vi "Two Color Cal Wait New Frame.vi"(0 "Notifier Name":string, 11 "Error In":errorcluster, 13 "Frames to Wait":u32) -> (15 "Error Out":errorcluster)   [LabVIEW 2016]
uses:
  Device Library/Cameras/Camera Controls/Generic Camera Actions.ctl
  Device Library/Cameras/Camera Controls/Camera IMAQ Key Info.ctl
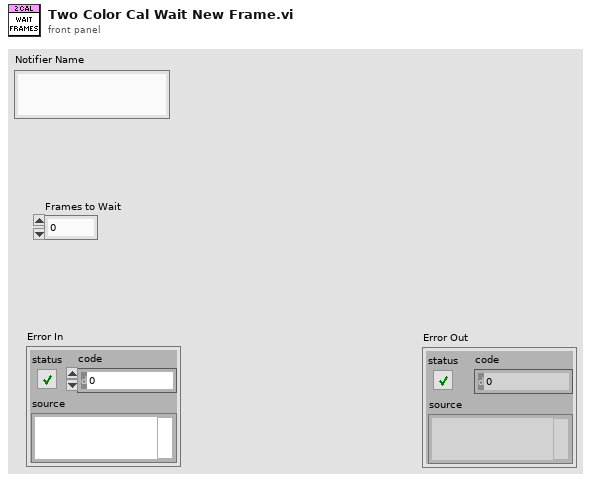
[diagram p1: front panel]
types:
  T1 = typedef "Generic Camera Actions.ctl" = enum16{"Status", "Live Preview", "Capture", "Abort", "Set Exposure Time (s)", "Get Exposure Time (s)", "Record Settings", "Set ROI", "Get ROI", "Defect Correction On/Off", "Cooler On/Off", "Fan On/Off", "Quti"}
  T2 = typedef "IMAQ Image.ctl" = refnum<image>
  T3 = typedef "Camera IMAQ Key Info.ctl" = cluster{"Frame":u32, "Sensor Height":i32, "Sensor Width":i32, "ROI Height":i32, "ROI Width":i32, "ROI Enable?":bool, "Bit per Pixel":u8}
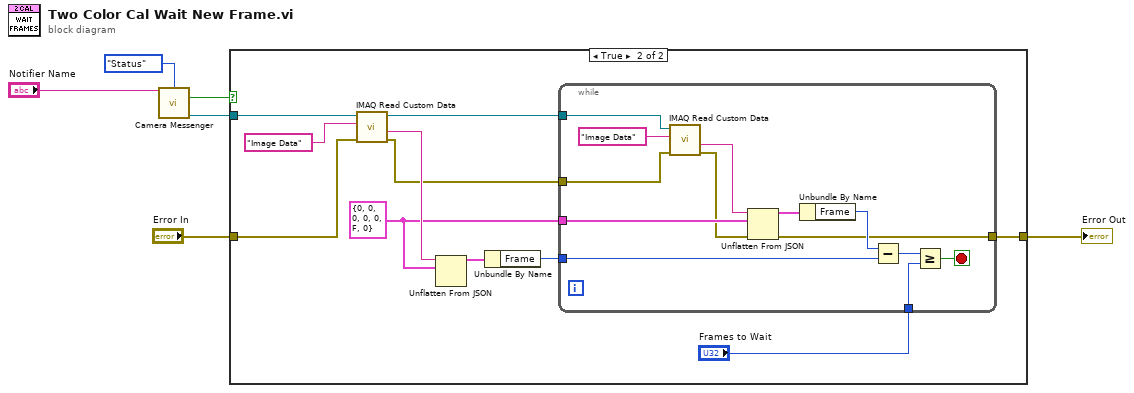
[diagram p0: block diagram]
diagram:
  n1 = call "Camera Messenger.vi"("Notifier Name"="Notifier Name", "General Camera Actions"=Generic_Camera_Actions."Status") -> ("Running?"=w3:bool, "Image Ref"=w5:T2)  [unwired: 8 in, 4 out]
  n2 = case shown="True" w3 {
    tunnel: w5 -> [_ w16]
    tunnel: [w7 w9] -> w2
    tunnel: "Error In" -> [w7 w8]
    frame False {
    }
    frame True {
      w14 = T3 {"Frame"=0, "Sensor Height"=0, "Sensor Width"=0, "ROI Height"=0, "ROI Width"=0, "ROI Enable?"=FALSE, "Bit per Pixel"=0} ("Camera IMAQ Key Info")
      n3 = call "IMAQ Read Custom Data"("error in (no error)"=w8, "Key"="Image Data", "Image"=w16) -> ("error out"=w10:errorcluster, "Custom Data Out"=w18:string, "Image (duplicate)"=w13:T2)  [unwired: 6 in]
      n4 = Unflatten From JSON(JSON string=w18, type and defaults=w14) -> (value=w15:T3)  [unwired: 5 in, 1 out]
      n5 = Unbundle By Name(w15) -> ("Frame"=w12:u32)
      n6 = while {
        tunnel: w13 -> [w27]
        tunnel: w14 -> [w28]
        tunnel: w12 -> [w25]
        tunnel: "Frames to Wait" -> [w23]
        tunnel: w10 -> [w21]
        tunnel: [w19] -> w9
        stop <- w22 stop-if-true
        n7 = call "IMAQ Read Custom Data"("error in (no error)"=w21, "Key"="Image Data", "Image"=w27) -> ("error out"=w20:errorcluster, "Custom Data Out"=w30:string)  [unwired: 6 in, 1 out]
        n8 = Unflatten From JSON(JSON string=w30, type and defaults=w28, error in (no error)=w20) -> (value=w31:T3, error out=w19:errorcluster)  [unwired: 4 in]
        n9 = Unbundle By Name(w31) -> ("Frame"=w26:u32)
        n10 = Subtract(x=w26, y=w25) -> (x-y=w24:u32)
        n11 = Greater Or Equal?(x=w24, y=w23) -> (x >= y?=w22:bool)
      }
    }
  }
  "Error Out" <- w2
